vi "CMN_Cali.vi"(11 "Enum":T1(ring)=enum."CF_Z_Bridge") -> ()   [LabVIEW 2016]
uses:
  <vilib>/Utility/file.llb/Write To Spreadsheet File (DBL).vi
panel:
  out "appended array":dbl[](array[numeric])
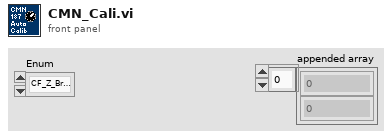
[diagram p1: front panel]
types:
  T1 = enum16{"CF", "CF_Z_Bridge", "MNK", "MNK_Z_Bridge"}
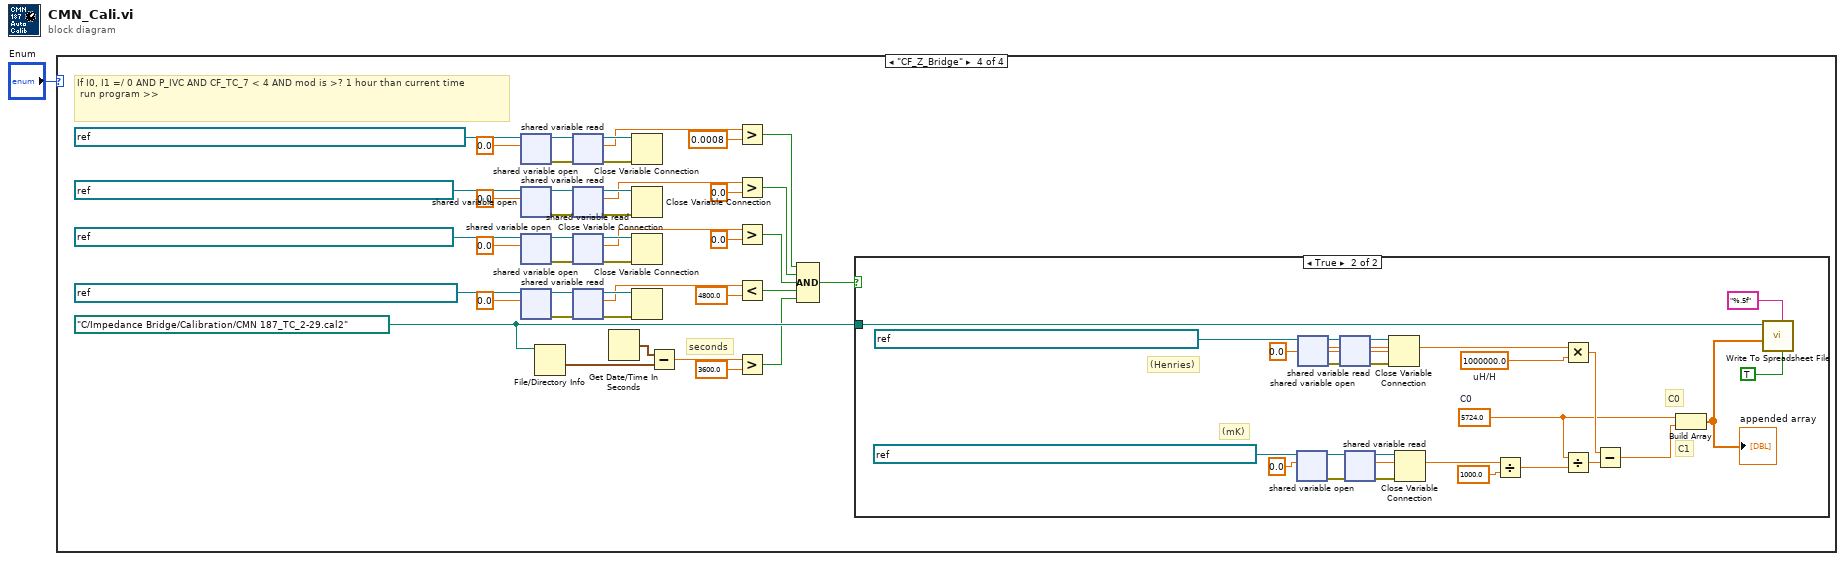
[diagram p0: block diagram]
diagram:
  n1 = case shown="\"CF_Z_Bridge\"" "Enum" {
    frame "CF", Default {
    }
    frame "MNK" {
    }
    frame "MNK_Z_Bridge" {
    }
    frame "CF_Z_Bridge" {
      w44 = path "C:/Impedance Bridge/Calibration/CMN 187_TC_2-29.cal2" ("file path (dialog if empty)")
      # "seconds"
      # "If I0, I1 =/ 0 AND P_IVC AND CF_TC_7 < 4 AND mod is >? 1 hour than current time\n run program >>"
      n2 = shared-variable-open(refnum<k21> "ni.var.psp://housesoftheholy/Leiden CF900/Leiden CF FP/CF FP MG3" ("shared variable refnum in"), 0.0 ("y")) -> (w27:refnum<k21>, w25:errorcluster)  [unwired: 2 in]
      n3 = shared-variable-open(refnum<k21> "ni.var.psp://housesoftheholy/Leiden CF900/Leiden CF TC/CF TC I0" ("shared variable refnum in"), 0.0 ("y")) -> (w43:refnum<k21>, w41:errorcluster)  [unwired: 2 in]
      n4 = shared-variable-open(refnum<k21> "ni.var.psp://housesoftheholy/Leiden CF900/Leiden CF TC/CF TC I1" ("shared variable refnum in"), 0.0 ("y")) -> (w37:refnum<k21>, w35:errorcluster)  [unwired: 2 in]
      n5 = shared-variable-open(refnum<k21> "ni.var.psp://housesoftheholy/Leiden CF900/Leiden CF TC/CF TC T7" ("shared variable refnum in"), 0.0 ("y")) -> (w10:refnum<k21>, w12:errorcluster)  [unwired: 2 in]
      n6 = File/Directory Info(path=w44) -> (last mod=w6:timestamp)  [unwired: 1 in, 6 out]
      n7 = shared-variable-read(w27, w25) -> (w26:refnum<k21>, w24:errorcluster, w21:dbl)  [unwired: 1 out]
      n8 = shared-variable-read(w43, w41) -> (w42:refnum<k21>, w40:errorcluster, w31:dbl)  [unwired: 1 out]
      n9 = shared-variable-read(w37, w35) -> (w36:refnum<k21>, w34:errorcluster, w28:dbl)  [unwired: 1 out]
      n10 = shared-variable-read(w10, w12) -> (w11:refnum<k21>, w13:errorcluster, w9:dbl)  [unwired: 1 out]
      n11 = Get Date/Time In Seconds() -> (seconds since 1Jan1904=w7:timestamp)
      n12 = Close Variable Connection(8:w24, 11:w26) -> ()  [unwired: 1 out]
      n13 = Close Variable Connection(8:w40, 11:w42) -> ()  [unwired: 1 out]
      n14 = Close Variable Connection(8:w34, 11:w36) -> ()  [unwired: 1 out]
      n15 = Close Variable Connection(8:w13, 11:w11) -> ()  [unwired: 1 out]
      n16 = Subtract(x=w7, y=w6) -> (x-y=w5:dbl)
      n17 = Greater?(x=w21, y=0.0008) -> (0:w19:bool)
      n18 = Greater?(x=w31, y=0.0) -> (0:w18:bool)
      n19 = Greater?(x=w28, y=0.0) -> (0:w17:bool)
      n20 = Less?(x=w9, y=4800.0) -> (x < y?=w2:bool)
      n21 = Greater?(x=w5, y=3600.0) -> (0:w3:bool)
      n22 = Compound Arithmetic op=AND(w19, w18, w17, w2, w3) -> (w16:bool)
      n23 = case shown="True" w16 {
        tunnel: w44 -> [_ w48]
        frame False {
        }
        frame True {
          w68 = 1000000.0  # uH/H
          w66 = 5724.0  # C0
          # "C0"
          # "C1"
          # "(Henries)"
          # "(mK)"
          n24 = shared-variable-open(refnum<k21> "ni.var.psp://housesoftheholy/Leiden CF900/Leiden CF TC/CF TC T7" ("shared variable refnum in"), 0.0 ("y")) -> (w49:refnum<k21>, w51:errorcluster)  [unwired: 2 in]
          n25 = shared-variable-open(refnum<k21> "ni.var.psp://housesoftheholy/Leiden CF900/CF_TC_Z_R0" ("shared variable refnum in"), 0.0 ("y")) -> (w61:refnum<k21>, w59:errorcluster)  [unwired: 2 in]
          n26 = shared-variable-read(w61, w59) -> (w60:refnum<k21>, w58:errorcluster, w55:dbl)  [unwired: 1 out]
          n27 = shared-variable-read(w49, w51) -> (w50:refnum<k21>, w52:errorcluster, w47:dbl)  [unwired: 1 out]
          n28 = Close Variable Connection(8:w58, 11:w60) -> ()  [unwired: 1 out]
          n29 = Close Variable Connection(8:w52, 11:w50) -> ()  [unwired: 1 out]
          n30 = Divide(x=w47, y=1000.0) -> (x/y=w45:dbl)
          n31 = Multiply(x=w55, y=w68) -> (x*y=w67:dbl)
          n32 = Divide(x=w66, y=w45) -> (x/y=w69:dbl)
          n33 = Subtract(x=w67, y=w69) -> (x-y=w65:dbl)
          n34 = Build Array(w66, w65) -> (w64:dbl[])
          "appended array" <- w64
          n35 = call-poly <vilib>:"Write To Spreadsheet File.vi"("transpose? (no:F)"=TRUE, "format (%.3f)"="%.5f", "1D data"=w64, "file path (dialog if empty)"=w48) -> ()  [unwired: 4 in, 1 out]
        }
      }
    }
  }
